vi "Ascii_Char.vi"(1 "number":u8) -> (0 "ascii char":string)   [LabVIEW 2017]
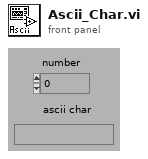
[diagram p1: front panel]
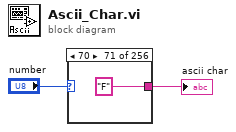
[diagram p0: block diagram]
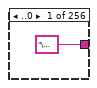
[diagram p2: hidden frame]
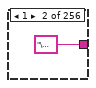
[diagram p3: hidden frame]
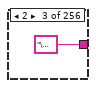
[diagram p4: hidden frame]
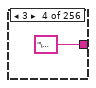
[diagram p5: hidden frame]
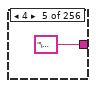
[diagram p6: hidden frame]
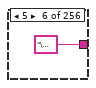
[diagram p7: hidden frame]
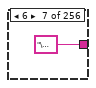
[diagram p8: hidden frame]
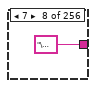
[diagram p9: hidden frame]
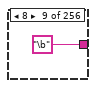
[diagram p10: hidden frame]
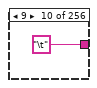
[diagram p11: hidden frame]
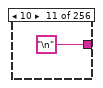
[diagram p12: hidden frame]
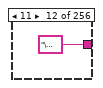
[diagram p13: hidden frame]
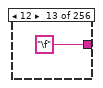
[diagram p14: hidden frame]
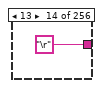
[diagram p15: hidden frame]
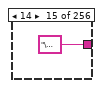
[diagram p16: hidden frame]
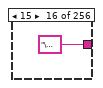
[diagram p17: hidden frame]
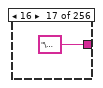
[diagram p18: hidden frame]
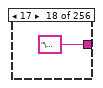
[diagram p19: hidden frame]
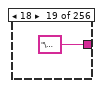
[diagram p20: hidden frame]
diagram:
  n1 = case shown="70" "number" {
    tunnel: ["\u0000" "\u0001" "\u0002" "\u0003" "\u0004" "\u0005" "\u0006" "\u0007" "\b" "\t" "\n" "\u000b" "\f" "\r" "\u000e" "\u000f" "\u0010" "\u0011" "\u0012" "\u0013" "\u0014" "\u0015" "\u0016" "\u0017" "\u0018" "\u0019" "\u001a" "\u001b" "\u001c" "\u001d" "\u001e" "\u001f" " " "!" "\"" "#" "$" "%" "&" "'" "(" ")" "*" "+" "," "-" "." "/" "0" "1" "2" "3" "4" "5" "6" "7" "8" "9" ":" ";" "<" "=" ">" "?" "@" "A" "B" "C" "D" "E" "F" "G" "H" "I" "J" "K" "L" "M" "N" "O" "P" "Q" "R" "S" "T" "U" "V" "W" "X" "Y" "Z" "[" "\\" "]" "^" "_" "`" "a" "b" "c" "d" "e" "f" "g" "h" "i" "j" "k" "l" "m" "n" "o" "p" "q" "r" "s" "t" "u" "v" "w" "x" "y" "z" "{" "|" "}" "~" "" "€" "" "‚" "ƒ" "„" "…" "†" "‡" "ˆ" "‰" "Š" "‹" "Œ" "" "Ž" "" "" "‘" "’" "“" "”" "•" "–" "—" "˜" "™" "š" "›" "œ" "" "ž" "Ÿ" " " "¡" "¢" "£" "¤" "¥" "¦" "§" "¨" "©" "ª" "«" "¬" "­" "®" "¯" "°" "±" "²" "³" "´" "µ" "¶" "·" "¸" "¹" "º" "»" "¼" "½" "¾" "¿" "À" "Á" "Â" "Ã" "Ä" "Å" "Æ" "Ç" "È" "É" "Ê" "Ë" "Ì" "Í" "Î" "Ï" "Ð" "Ñ" "Ò" "Ó" "Ô" "Õ" "Ö" "×" "Ø" "Ù" "Ú" "Û" "Ü" "Ý" "Þ" "ß" "à" "á" "â" "ã" "ä" "å" "æ" "ç" "è" "é" "ê" "ë" "ì" "í" "î" "ï" "ð" "ñ" "ò" "ó" "ô" "õ" "ö" "÷" "ø" "ù" "ú" "û" "ü" "ý" "þ" "ÿ"] -> w1
    frame ..0 {
    }
    frame 1 {
    }
    frame 2 {
    }
    frame 3 {
    }
    frame 4 {
    }
    frame 5 {
    }
    frame 6 {
    }
    frame 7 {
    }
    frame 8 {
    }
    frame 9 {
    }
    frame 10 {
    }
    frame 11 {
    }
    frame 12 {
    }
    frame 13 {
    }
    frame 14 {
    }
    frame 15 {
    }
    frame 16 {
    }
    frame 17 {
    }
    frame 18 {
    }
    frame 19 {
    }
    frame 20 {
    }
    frame 21 {
    }
    frame 22 {
    }
    frame 23 {
    }
    frame 24 {
    }
    frame 25 {
    }
    frame 26 {
    }
    frame 27 {
    }
    frame 28 {
    }
    frame 29 {
    }
    frame 30 {
    }
    frame 31 {
    }
    frame 32 {
    }
    frame 33 {
    }
    frame 34 {
    }
    frame 35 {
    }
    frame 36 {
    }
    frame 37 {
    }
    frame 38 {
    }
    frame 39 {
    }
    frame 40 {
    }
    frame 41 {
    }
    frame 42 {
    }
    frame 43 {
    }
    frame 44 {
    }
    frame 45 {
    }
    frame 46 {
    }
    frame 47 {
    }
    frame 48 {
    }
    frame 49 {
    }
    frame 50 {
    }
    frame 51 {
    }
    frame 52 {
    }
    frame 53 {
    }
    frame 54 {
    }
    frame 55 {
    }
    frame 56 {
    }
    frame 57 {
    }
    frame 58 {
    }
    frame 59 {
    }
    frame 60 {
    }
    frame 61 {
    }
    frame 62 {
    }
    frame 63 {
    }
    frame 64 {
    }
    frame 65 {
    }
    frame 66 {
    }
    frame 67 {
    }
    frame 68 {
    }
    frame 69 {
    }
    frame 70 {
    }
    frame 71 {
    }
    frame 72 {
    }
    frame 73 {
    }
    frame 74 {
    }
    frame 75 {
    }
    frame 76 {
    }
    frame 77 {
    }
    frame 78 {
    }
    frame 79 {
    }
    frame 80 {
    }
    frame 81 {
    }
    frame 82 {
    }
    frame 83 {
    }
    frame 84 {
    }
    frame 85 {
    }
    frame 86 {
    }
    frame 87 {
    }
    frame 88 {
    }
    frame 89 {
    }
    frame 90 {
    }
    frame 91 {
    }
    frame 92 {
    }
    frame 93 {
    }
    frame 94 {
    }
    frame 95 {
    }
    frame 96 {
    }
    frame 97 {
    }
    frame 98 {
    }
    frame 99 {
    }
    frame 100 {
    }
    frame 101 {
    }
    frame 102 {
    }
    frame 103 {
    }
    frame 104 {
    }
    frame 105 {
    }
    frame 106 {
    }
    frame 107 {
    }
    frame 108 {
    }
    frame 109 {
    }
    frame 110 {
    }
    frame 111 {
    }
    frame 112 {
    }
    frame 113 {
    }
    frame 114 {
    }
    frame 115 {
    }
    frame 116 {
    }
    frame 117 {
    }
    frame 118 {
    }
    frame 119 {
    }
    frame 120 {
    }
    frame 121 {
    }
    frame 122 {
    }
    frame 123 {
    }
    frame 124 {
    }
    frame 125 {
    }
    frame 126 {
    }
    frame 127 {
    }
    frame 128 {
    }
    frame 129 {
    }
    frame 130 {
    }
    frame 131 {
    }
    frame 132 {
    }
    frame 133 {
    }
    frame 134 {
    }
    frame 135 {
    }
    frame 136 {
    }
    frame 137 {
    }
    frame 138 {
    }
    frame 139 {
    }
    frame 140 {
    }
    frame 141 {
    }
    frame 142 {
    }
    frame 143 {
    }
    frame 144 {
    }
    frame 145 {
    }
    frame 146 {
    }
    frame 147 {
    }
    frame 148 {
    }
    frame 149 {
    }
    frame 150 {
    }
    frame 151 {
    }
    frame 152 {
    }
    frame 153 {
    }
    frame 154 {
    }
    frame 155 {
    }
    frame 156 {
    }
    frame 157 {
    }
    frame 158 {
    }
    frame 159 {
    }
    frame 160 {
    }
    frame 161 {
    }
    frame 162 {
    }
    frame 163 {
    }
    frame 164 {
    }
    frame 165 {
    }
    frame 166 {
    }
    frame 167 {
    }
    frame 168 {
    }
    frame 169 {
    }
    frame 170 {
    }
    frame 171 {
    }
    frame 172 {
    }
    frame 173 {
    }
    frame 174 {
    }
    frame 175 {
    }
    frame 176 {
    }
    frame 177 {
    }
    frame 178 {
    }
    frame 179 {
    }
    frame 180 {
    }
    frame 181 {
    }
    frame 182 {
    }
    frame 183 {
    }
    frame 184 {
    }
    frame 185 {
    }
    frame 186 {
    }
    frame 187 {
    }
    frame 188 {
    }
    frame 189 {
    }
    frame 190 {
    }
    frame 191 {
    }
    frame 192 {
    }
    frame 193 {
    }
    frame 194 {
    }
    frame 195 {
    }
    frame 196 {
    }
    frame 197 {
    }
    frame 198 {
    }
    frame 199 {
    }
    frame 200 {
    }
    frame 201 {
    }
    frame 202 {
    }
    frame 203 {
    }
    frame 204 {
    }
    frame 205 {
    }
    frame 206 {
    }
    frame 207 {
    }
    frame 208 {
    }
    frame 209 {
    }
    frame 210 {
    }
    frame 211 {
    }
    frame 212 {
    }
    frame 213 {
    }
    frame 214 {
    }
    frame 215 {
    }
    frame 216 {
    }
    frame 217 {
    }
    frame 218 {
    }
    frame 219 {
    }
    frame 220 {
    }
    frame 221 {
    }
    frame 222 {
    }
    frame 223 {
    }
    frame 224 {
    }
    frame 225 {
    }
    frame 226 {
    }
    frame 227 {
    }
    frame 228 {
    }
    frame 229 {
    }
    frame 230 {
    }
    frame 231 {
    }
    frame 232 {
    }
    frame 233 {
    }
    frame 234 {
    }
    frame 235 {
    }
    frame 236 {
    }
    frame 237 {
    }
    frame 238 {
    }
    frame 239 {
    }
    frame 240 {
    }
    frame 241 {
    }
    frame 242 {
    }
    frame 243 {
    }
    frame 244 {
    }
    frame 245 {
    }
    frame 246 {
    }
    frame 247 {
    }
    frame 248 {
    }
    frame 249 {
    }
    frame 250 {
    }
    frame 251 {
    }
    frame 252 {
    }
    frame 253 {
    }
    frame 254 {
    }
    frame 255.. {
    }
  }
  "ascii char" <- w1
